vi "Parse XML dateTime String.vi"(8 "error in (no error)":errorcluster, 10 "xml dateTime string":string) -> (0 "error out":errorcluster, 2 "Time Stamp":timestamp)   [LabVIEW 2013]
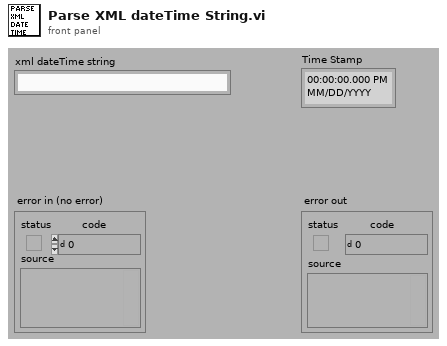
[diagram p1: front panel]
types:
  T1 = cluster{"second":i32, "minute":i32, "hour":i32, "day of month":i32, "month":i32, "year":i32, "day of week":i32, "day of year":i32, "is DST":i32}
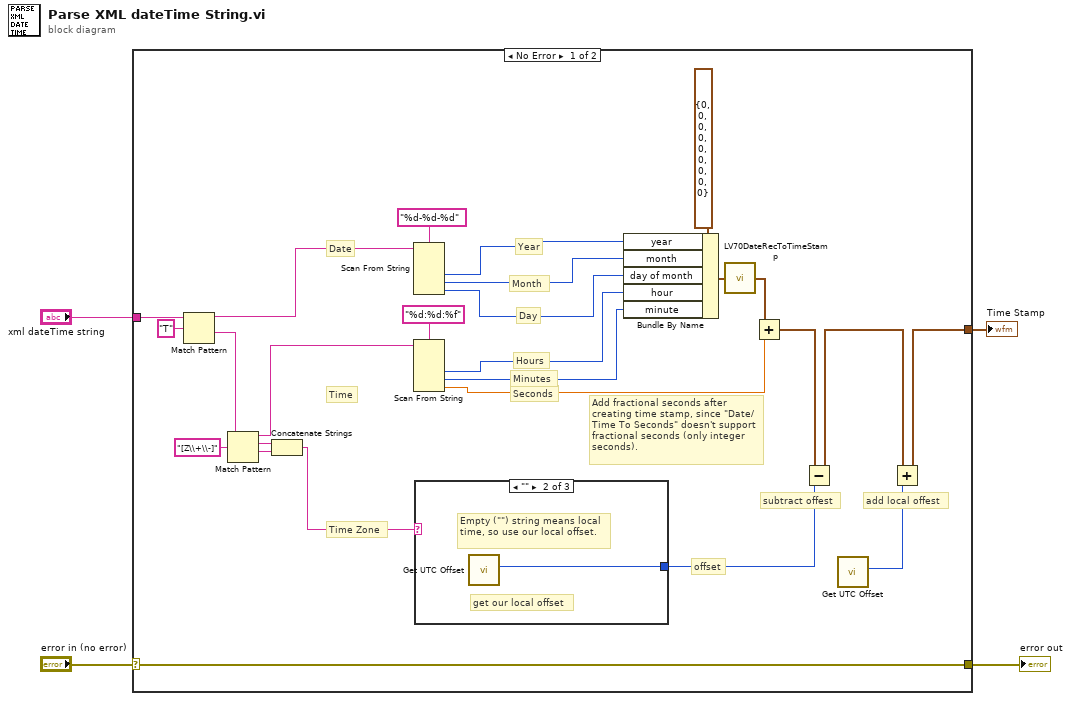
[diagram p0: block diagram]
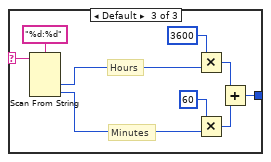
[diagram p3: hidden frame]
diagram:
  n1 = case shown="No Error" "error in (no error)" {
    selector: "error in (no error)" -> [w10 w41]
    tunnel: "xml dateTime string" -> [w30 _]
    tunnel: [w8 _] -> w2
    tunnel: [w10 w41] -> w3
    frame No Error {
      # "add local offest"
      # "Time Zone"
      # "Date"
      # "Time"
      # "offset"
      # "Add fractional seconds after creating time stamp, since \"Date/Time To Seconds\" doesn't support fractional seconds (only integer seconds)."
      # "Seconds"
      # "Minutes"
      # "Hours"
      # "Day"
      # "Month"
      # "Year"
      # "subtract offest"
      n2 = Match Pattern(string=w30, regular expression="T") -> (before substring=w23:string, after substring=w25:string)  [unwired: 1 in, 2 out]
      n3 = Match Pattern(string=w25, regular expression="[Z\\+\\-]") -> (before substring=w21:string, match substring=w27:string, after substring=w26:string)  [unwired: 1 in, 1 out]
      n4 = Concatenate Strings(w27, w26) -> (w11:string)
      n5 = Scan From String(format string="%d-%d-%d", input string=w23) -> (output 1=w18:i32, output 2=w17:i32, output 3=w16:i32)  [unwired: 5 in, 3 out]
      n6 = Scan From String(format string="%d:%d:%f", input string=w21) -> (output 1=w15:i32, output 2=w14:i32, output 3=w7:dbl)  [unwired: 5 in, 3 out]
      n7 = case shown="\"\"" w11 {
        selector: w11 -> [_ _ w32]
        tunnel: [_ w31 w33] -> w12
        frame "Z", "z" {
          # "\"Z\" means UTC time. No offset"
        }
        frame "" {
          # "get our local offset"
          # "Empty (\"\") string means local time, so use our local offset."
          n8 = call "Get UTC Offset.vi"() -> ("UTC Offset (seconds)"=w31:i32)  [unwired: 10 in, 1 out]
        }
        frame Default {
          # "Hours"
          # "Minutes"
          n9 = Scan From String(format string="%d:%d", input string=w32) -> (output 1=w39:i32, output 2=w36:i32)  [unwired: 4 in, 3 out]
          n10 = Multiply(x=3600 ("y"), y=w39) -> (x*y=w35:i32)
          n11 = Multiply(x=60 ("y"), y=w36) -> (x*y=w34:i32)
          n12 = Add(x=w35, y=w34) -> (x+y=w33:i32)
        }
      }
      n13 = Bundle By Name(cluster=T1 {"second"=0, "minute"=0, "hour"=0, "day of month"=0, "month"=0, "year"=0, "day of week"=0, "day of year"=0, "is DST"=0} ("date time rec"), "year"=w18, "month"=w17, "day of month"=w16, "hour"=w15, "minute"=w14) -> (w19:T1)
      n14 = call <vilib>:"LV70DateRecToTimeStamp.vi"("date time rec"=w19) -> ("Time Stamp"=w13:timestamp)
      n15 = Add(x=w13, y=w7) -> (x+y=w6:timestamp)
      n16 = Subtract(x=w6, y=w12) -> (x-y=w5:timestamp)
      n17 = call "Get UTC Offset.vi"() -> ("UTC Offset (seconds)"=w9:i32)  [unwired: 10 in, 1 out]
      n18 = Add(x=w5, y=w9) -> (x+y=w8:timestamp)
    }
    frame Error {
    }
  }
  "error out" <- w3
  "Time Stamp" <- w2
